vi "Read Waveform Type.vi"(8 "error in (no error)":errorcluster, 11 "Waveform Type Message in":refnum<class "Waveform Type Message.lvclass">) -> (0 "error out":errorcluster, 2 "Waveform Type":T1, 3 "Waveform Type Message out":refnum<class "Waveform Type Message.lvclass">)   [LabVIEW 2011, in "Waveform Type Message.lvclass"]
uses:
  Waveform Type Message.lvclass
  Controls/Waveform Type.ctl
  Waveform Type Message.lvclass/Waveform Type Message.ctl
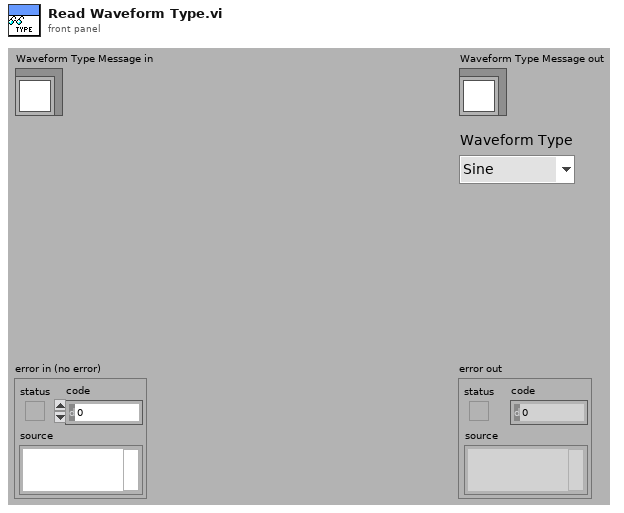
[diagram p1: front panel]
types:
  T1 = typedef "Waveform Type.ctl" = enum16{"Sine", "Square", "Triangle"}
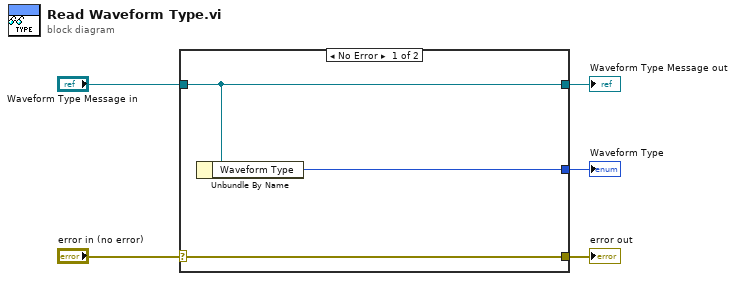
[diagram p0: block diagram]
diagram:
  n1 = case shown="No Error" "error in (no error)" {
    selector: "error in (no error)" -> [w8 w9]
    tunnel: [w8 w9] -> w4
    tunnel: [w7 w10] -> w2
    tunnel: "Waveform Type Message in" -> [w7 w10]
    tunnel: [w6 _] -> w1
    frame No Error {
      n2 = Unbundle By Name(w7) -> ("Waveform Type"=w6:T1)
    }
    frame Error {
    }
  }
  "error out" <- w4
  "Waveform Type Message out" <- w2
  "Waveform Type" <- w1
